vi "setEncoderToZero.vi"(2 "error in (no error)":errorcluster, 3 "VISA resource name":refnum<visa-resource-name>) -> (0 "error out":errorcluster, 1 "VISA resource name out":refnum<visa-resource-name>)   [LabVIEW 2020]
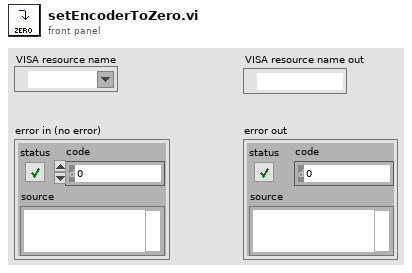
[diagram p1: front panel]
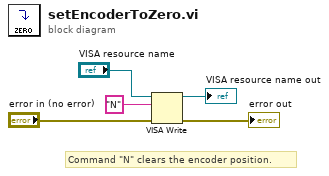
[diagram p0: block diagram]
diagram:
  # "Command \"N\" clears the encoder position."
  n1 = VISA Write(VISA resource name="VISA resource name", write buffer="N", error in (no error)="error in (no error)") -> (VISA resource name out=→"VISA resource name out":refnum<visa-resource-name>, error out=→"error out":errorcluster)  [unwired: 1 out]
